vi "FPGAmain_5782_IQ_PID.vi"() -> ()   [LabVIEW 2018]
uses:
  FPGA/DataMode.ctl
  FPGA/Input_5782/5782_Fast_PID_states.ctl
  FPGA/Feed forward/FeedForwardState.ctl
  FPGA/Feed forward/FeedForwardProcessingState.ctl
  <vilib>/Platform/TimedLoop/XDataNode/timing_clust.ctl
  <vilib>/Platform/TimedLoop/XDataNode/nitl_modes.ctl
  <vilib>/Platform/TimedLoop/XDataNode/wakeup.ctl
  <vilib>/rvi/Emulation/niFpgaSctlEmulationGetInTimedLoop.vi
  <vilib>/rvi/Emulation/niFpgaEmulationReportErrorSimple.vi
  <vilib>/rvi/Emulation/niFpgaGetClockAttributes.vi
  <vilib>/rvi/Emulation/niFpgaCriticalErrorInLSC.vi
  <vilib>/rvi/Emulation/niFpgaProcessEmulError.vi
  <vilib>/rvi/Emulation/niFpgaEmulationIsFPGAContextNoSignature.vi
  <vilib>/rvi/errors/niFpgaSetErrorForExecOnDevCompSimple.vi
  <vilib>/rvi/eio/common/nirviEmuReportErrorAndStop.vi
  <vilib>/rvi/DataTransferAndStorage/Container/Common/niFpgaContainerGetUniqueNameForEmu.vi
  <vilib>/rvi/FIFO/Fifo_Resource/nirvififoEmulationSetSize.vi
  <vilib>/rvi/FIFO/Fifo_Resource/nirviFifoEmulationQueueMgr.vi
  <instcachedir>/0/nirviFifoEmulationQueueMgr_E5CAEC123FF24DC58D834DCA3CDAA9B5.lvgen/nirviFifoEmulationQueueMgr_E5CAEC123FF24DC58D834DCA3CDAA9B5_015.vi
  <vilib>/rvi/FIFO/Fifo_Resource/nirvififoEmulationDetermineInputValidOut.vi
  <vilib>/rvi/FIFO/Fifo_Resource/nirvififoEmulationCreateLock.vi
  <vilib>/rvi/FIFO/Fifo_Resource/nirvififoEmulationObtainLock.vi
  <vilib>/rvi/FIFO/Fifo_Resource/nirvififoEmulationReleaseLock.vi
  <vilib>/rvi/occurrence/nirviWaitOnOccurrenceBase.vi
  <vilib>/rvi/errors/nirviReportUnexpectedCaseInternalError.vi
  <vilib>/rvi/errors/nirviReportUnexpectedCaseInternalError (U32).vi
  <vilib>/rvi/Memory/Memory_Emulation/niFpgaMemoryEmulationCacheClearOnFirstRun.vi
  <vilib>/rvi/Memory/Memory_Emulation/nirvimemoryEmulationManagerCache_MakeExclusive.vi
  <vilib>/rvi/Memory/Memory_Emulation/niFpgaMemoryEmulationValidateCache.vi
  <vilib>/rvi/Memory/Memory_Emulation/nirvimemoryEmulationManagerCache_InsertValue.vi
  <vilib>/Utility/error.llb/Clear Errors.vi
  <vilib>/rvi/Memory/Memory_Emulation/nirvimemoryEmulationManagerCache_ReleaseExclusive.vi
  <vilib>/rvi/Memory/Memory_Emulation/nirvimemoryEmulationManagerCache_GetValue.vi
  <vilib>/rvi/Memory/Memory_Emulation/nirvimemoryEmulationManagerCache_SetValue.vi
  <vilib>/rvi/eio/common/nirviEmuTemplateMethod_errors.vi
  <instcachedir>/0/nirviFifoEmulationQueueMgr_E5CAEC123FF24DC58D834DCA3CDAA9B5.lvgen/nirviFifoEmulationQueueMgr_E5CAEC123FF24DC58D834DCA3CDAA9B5_018.vi
  <vilib>/rvi/interface/RandomDataEmulation/niFpgaRandomDataHandleErrors.vi
  <instcachedir>/0/nirviFifoEmulationQueueMgr_E5CAEC123FF24DC58D834DCA3CDAA9B5.lvgen/nirviFifoEmulationQueueMgr_E5CAEC123FF24DC58D834DCA3CDAA9B5_003.vi
  <instcachedir>/0/nirviFifoEmulationQueueMgr_E5CAEC123FF24DC58D834DCA3CDAA9B5.lvgen/nirviFifoEmulationQueueMgr_E5CAEC123FF24DC58D834DCA3CDAA9B5_017.vi
  <vilib>/rvi/interface/RandomDataEmulation/nirviRandomDataMultiElementFPGAFIFO.vi
  <instcachedir>/0/nirviRandomDataMultiElementFPGAFIFO_6740B454F3C245F78F76ED91F73FD8DB.lvgen/nirviRandomDataMultiElementFPGAFIFO_6740B454F3C245F78F76ED91F73FD8DB_000.vi
  <instrlib>/_niInstr/Basic Elements/v1/FPGA/Private/Count Down U8.vi
  <vilib>/rvi/Memory/Memory_Emulation/nirvimemoryFastEmulation.vi
  <vilib>/rvi/Memory/Memory_Emulation/nirvimemoryEmulation.vi
  <vilib>/Platform/TimedLoop/XDataNode/XDataNode.xnode
  <vilib>/rvi/FXPMathLib/FxpInterpret/XNode/nifxpmath_Interpret.xnode
  <vilib>/rvi/DataTransferAndStorage/Container/XNode/niFpgaContainer.xnode
  <vilib>/rvi/FIFO/Fifo_Resource/nirvififoEmulationWrite.vi
  <vilib>/rvi/DataTransferAndStorage/Register/Emulation/niFpgaRegisterEmulation.vi
  <vilib>/eio/EIONode/EIONode.xnode
  <vilib>/rvi/FIFO/Fifo_Resource/nirvififoEmulationRead.vi
  <vilib>/rvi/interface/RandomDataEmulation/nirviRandomDataFpgaReadWriteTemplate.vi
  <vilib>/rvi/interface/RandomDataEmulation/nirviRandomDataFpgaMultiElementTemplate.vi
  <vilib>/Platform/TimedLoop/XDataNode/XDNodeRunTimeDep.lvlib
  <instrlib>/_niInstr/Basic Elements/v1/FPGA/niInstr Basic Elements v1 FPGA.lvlib
panel:
  in  "Ultra low speed transfer":bool
  out "5782 states":T1
  out "Read FF address":u32
  in  "Load FF":bool
  in  "Clear feedback buffers":bool
  in  "FF buffers manual":bool
  in  "Full speed transfer":bool
  in  "IO Module\\AO Data Sync":bool=TRUE
  in  "IO Module\\SPI Write Data":u16
  out "IO Module\\SPI Read Data":u8
  in  "IO Module\\SPI Read":bool
  in  "IO Module\\SPI Write":bool
  in  "IO Module\\SPI Address":u16
  in  "IO Module\\SPI Device":u8
  out "IO Module\\SPI Idle":bool
  in  "AM phase":fxp<+,64,64>
  in  "User Command Commit":bool
  in  "User Command":u8
  out "User Command Idle":bool
  out "User Command Status":u8
  in  "User Data 0":u8
  in  "User Data 1":u8
  out "PLL Locked":bool
  out "User Error":bool
  out "Configured?":bool
  in  "Continuous":bool
  in  "Record length":u16=4000 caption="Samples Per Trigger" min=1 step=1
  in  "Trigger Acquisition":bool
  out "IO Module\\Trigger Input":bool
  in  "Acquisition running":bool
  in  "Phase output":fxp<+,64,64>[](array[numeric])=[0.0, 0.0, 0.0, 0.0]
  in  "Simulated phase":fxp<+,64,64>[](array[numeric])=[0.0, 0.0]
  in  "Mode":T2
  in  "Phase input":fxp<+,64,64>[](array[numeric])=[0.0, 0.0, 0.0, 0.0, 0.0, 0.0, 0.0, 0.0, 0.0, 0.0, 0.0, 0.0, 0.0, 0.0, 0.0, 0.0]
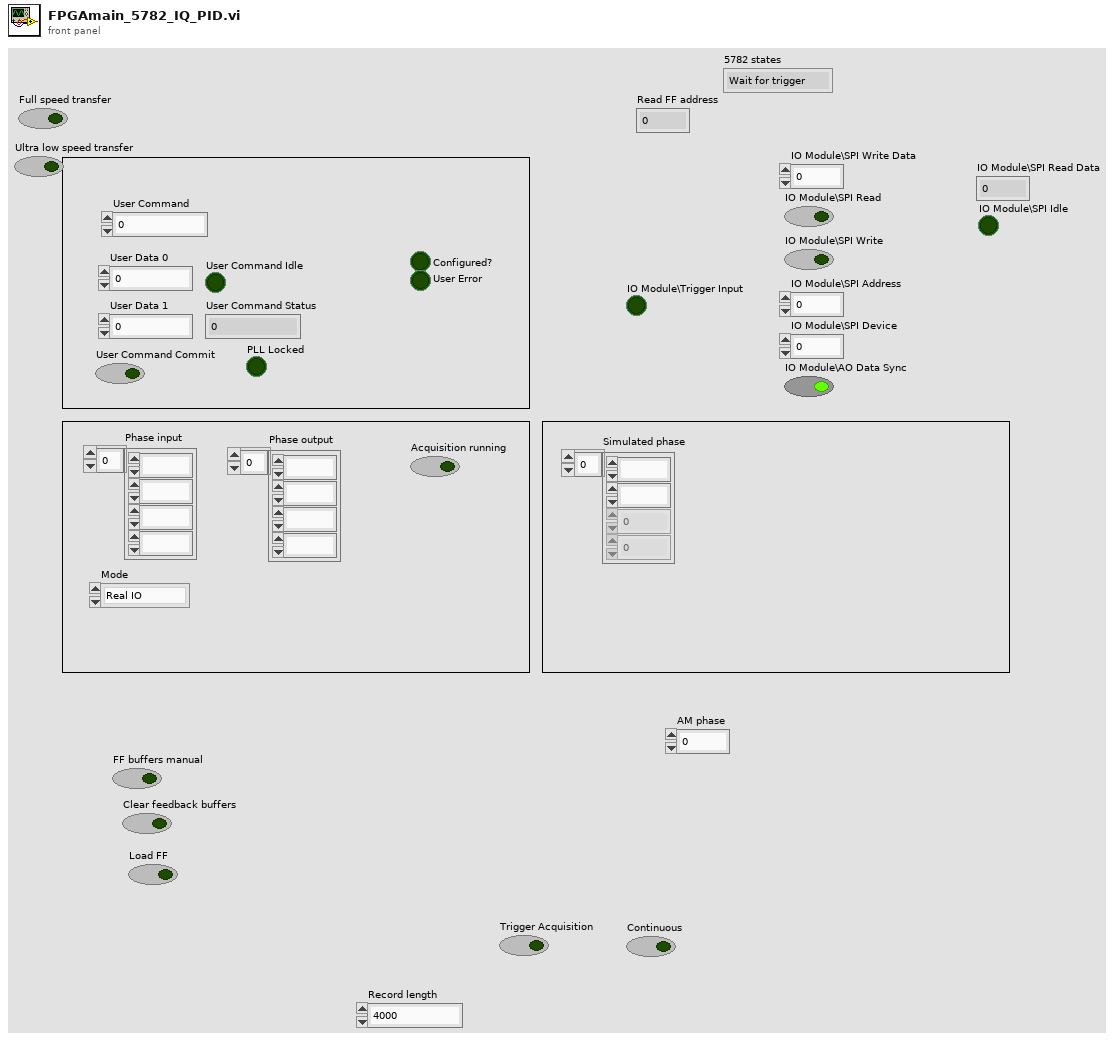
[diagram p1: front panel]
types:
  T1 = typedef "5782_Fast_PID_states.ctl" = enum8{"Wait for trigger", "Acquisition", "Send record length", "Wait for output", "Quiet period"}
  T2 = typedef "DataMode.ctl" = enum16{"Real IO", "Simulated"}
  T3 = typedef "FeedForwardProcessingState.ctl" = enum16{"Wait for trigger", "Processing", "Filtering", "Wait for reset"}
  T4 = typedef "FeedForwardState.ctl" = enum16{"Idle", "Wait for trigger", "Read FF", "Clear FF", "Wait for reset"}
  T5 = typedef "XDNodeRunTimeDep.lvlib/timing_clust.ctl" = cluster{"Expected End [f-1]":u64, "Actual End [f-1]":u64, "Finished Late? [f-1]":bool, "Expected End [i-1]":u64, "Actual End [i-1]":u64, "Finished Late? [i-1]":bool, "Expected Start [i]":u64, "Actual Start [i]":u64, "Expected Start [f]":u64, "Actual Start [f]":u64, "Source Name":string, "Structure Name":string, "Period":i64, "Deadline":i64, "Offset":i64, "Start":i64, "Priority":i32, "Timeout":i32, "Mode":T6, "Wakeup Reason":T7, "Error":errorcluster, "Source Type":string, "Secondary Source Type":string, "Global End Time":u64, "Global Start Time":u64, "Frame Duration":u64, "Iteration Duration":u64, "Assigned CPU":i32, "I/O Scan Engine Mode":u32}
  T6 = typedef "XDNodeRunTimeDep.lvlib/nitl_modes.ctl" = enum32{"No Change", "Process missed periods, maintain original phase", "Discard missed periods, maintain original phase", "Process missed periods, ignore original phase", "Discard missed periods, ignore original phase"}
  T7 = typedef "XDNodeRunTimeDep.lvlib/wakeup.ctl" = enum32{"Normal", "Aborted", "Asynchronous wakeup", "Timing source error", "Timed loop error", "Timeout"}
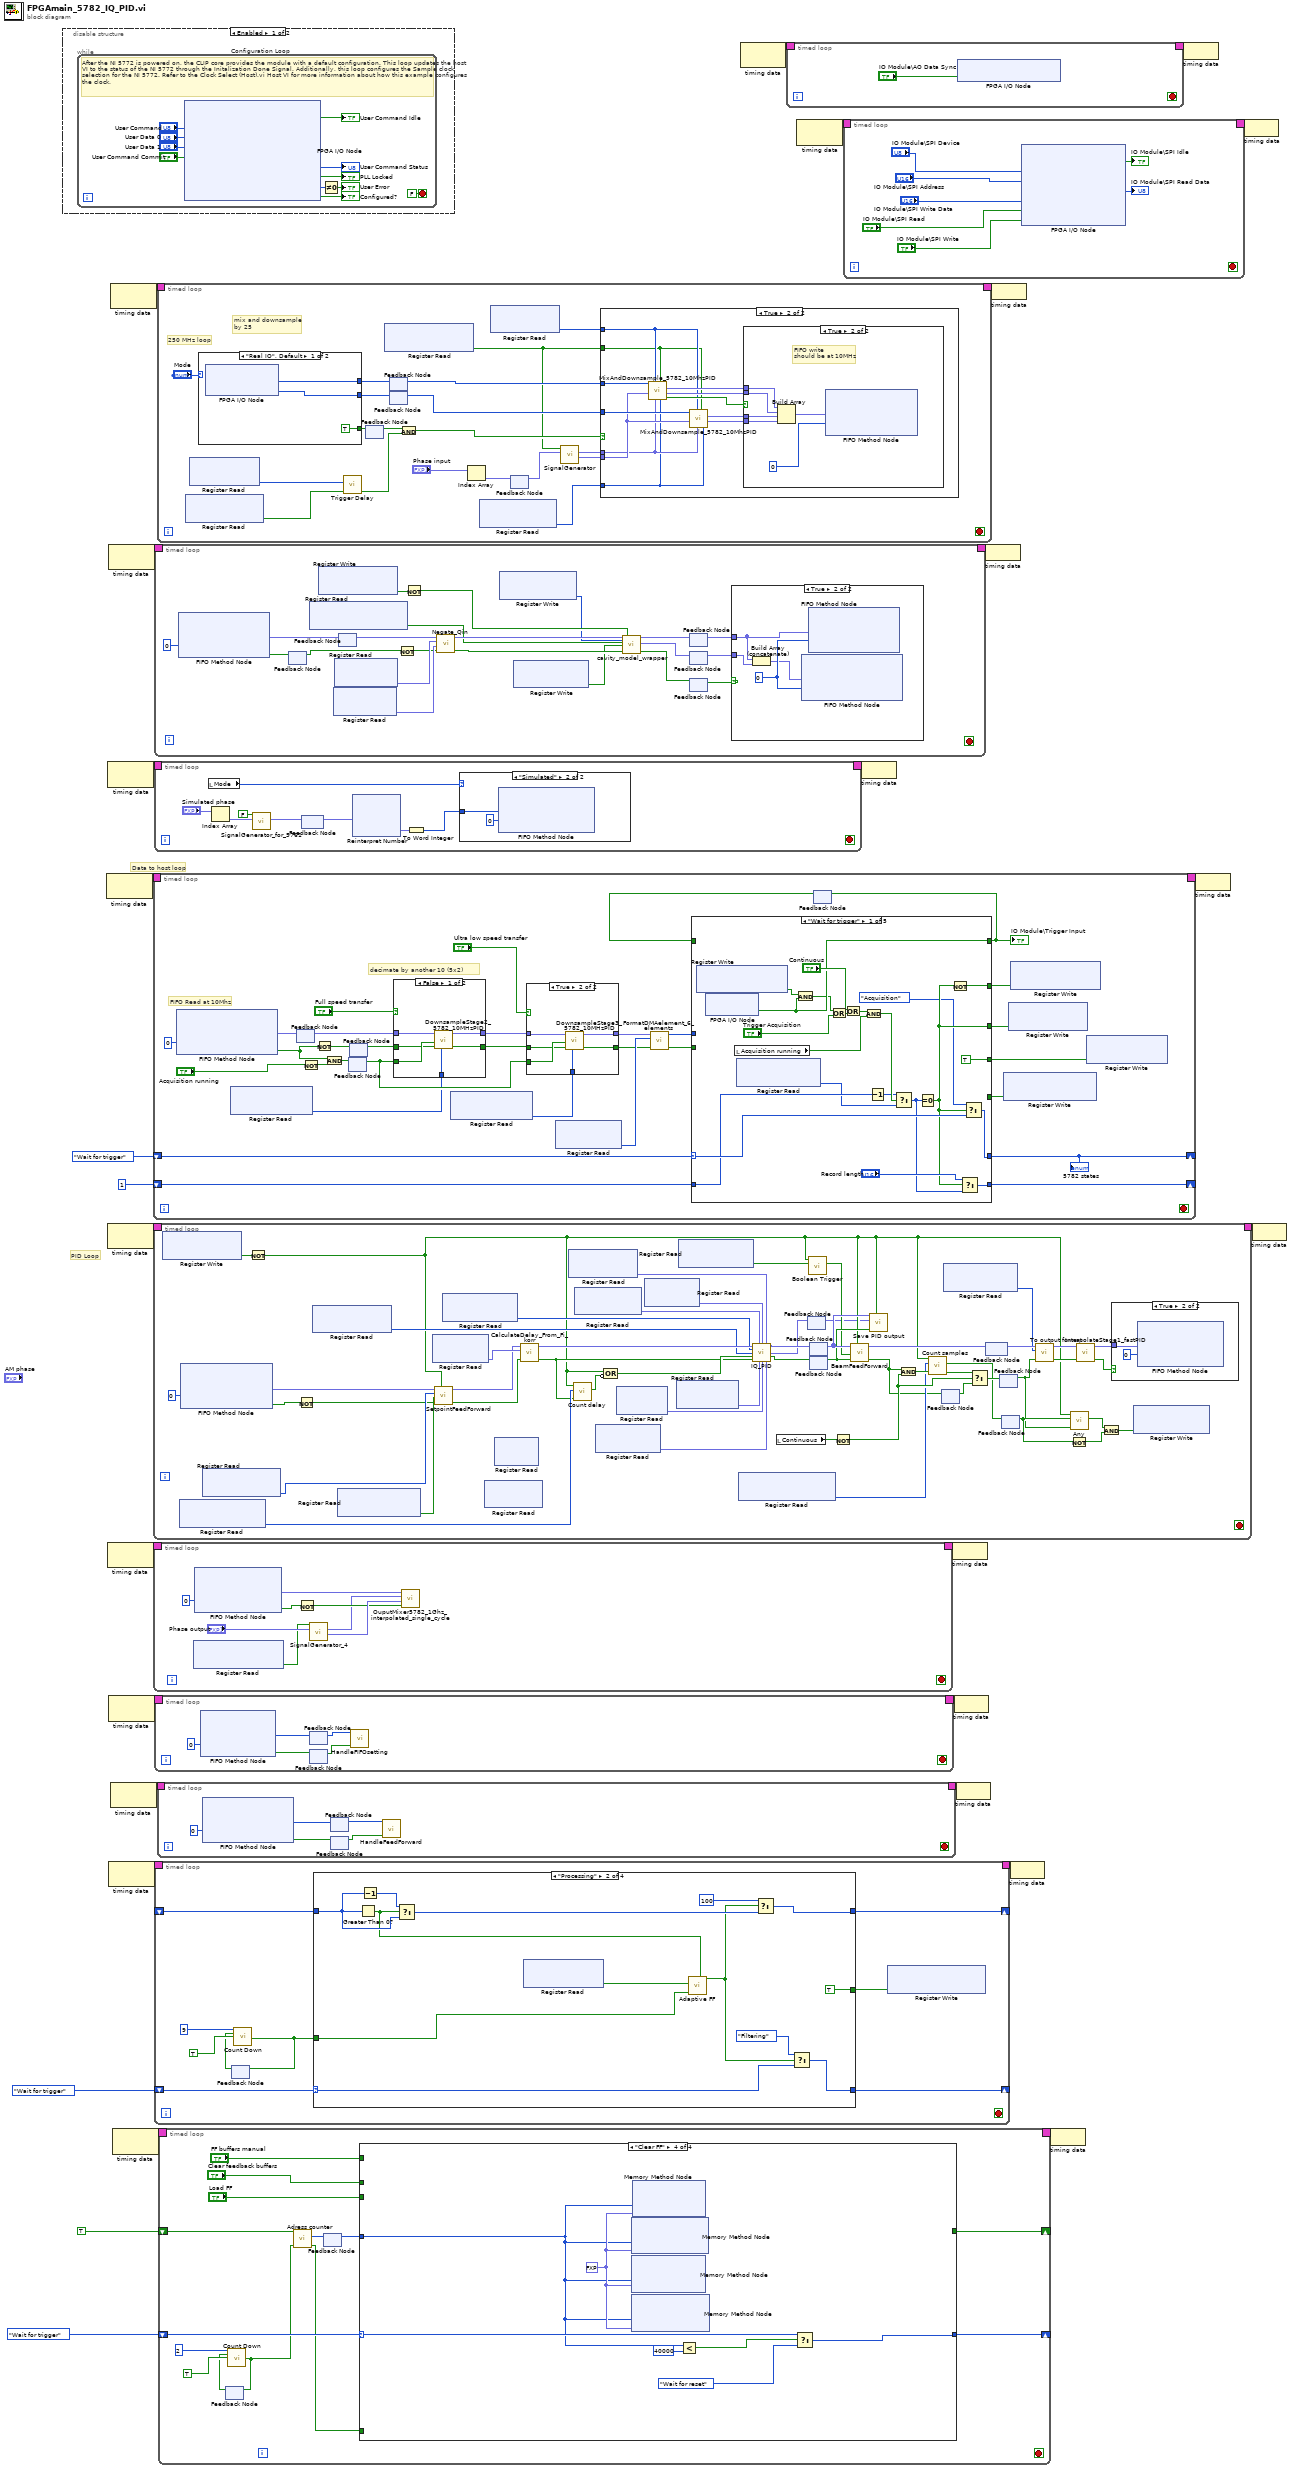
[diagram p0: block diagram]
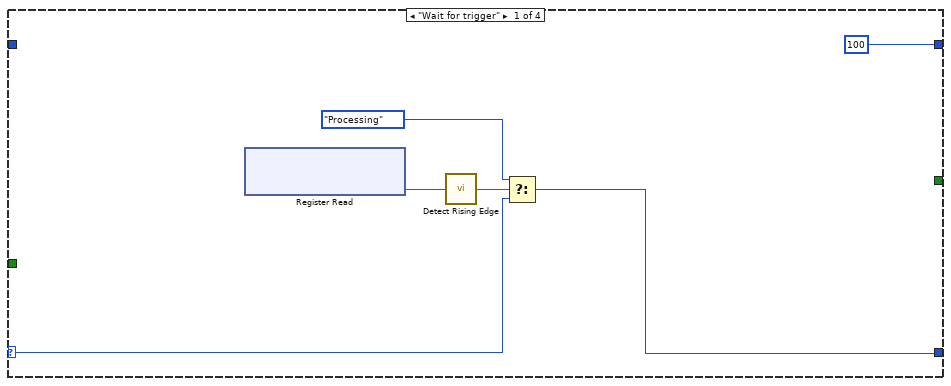
[diagram p2: hidden frame]
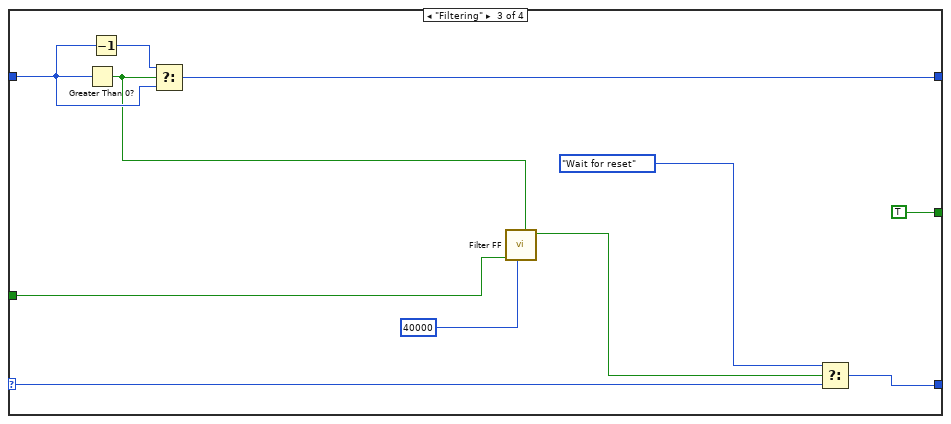
[diagram p3: hidden frame]
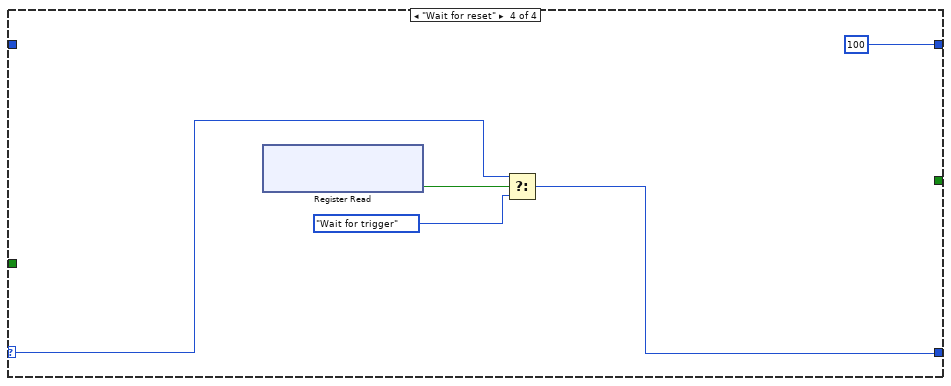
[diagram p4: hidden frame]
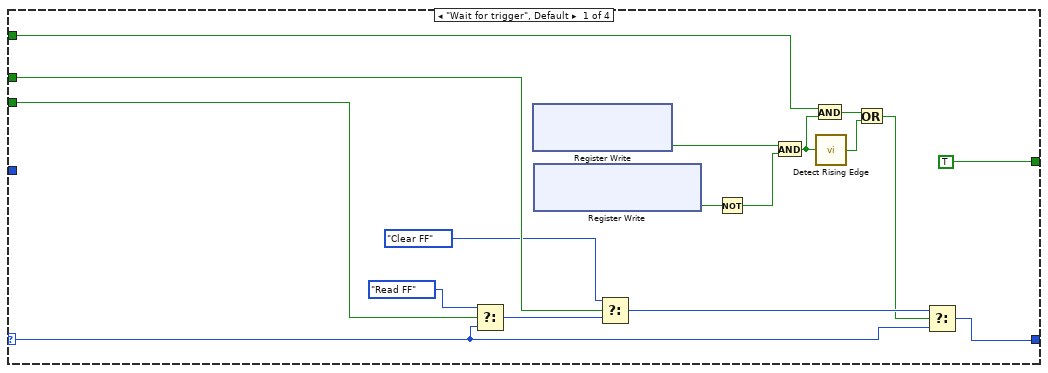
[diagram p5: hidden frame]
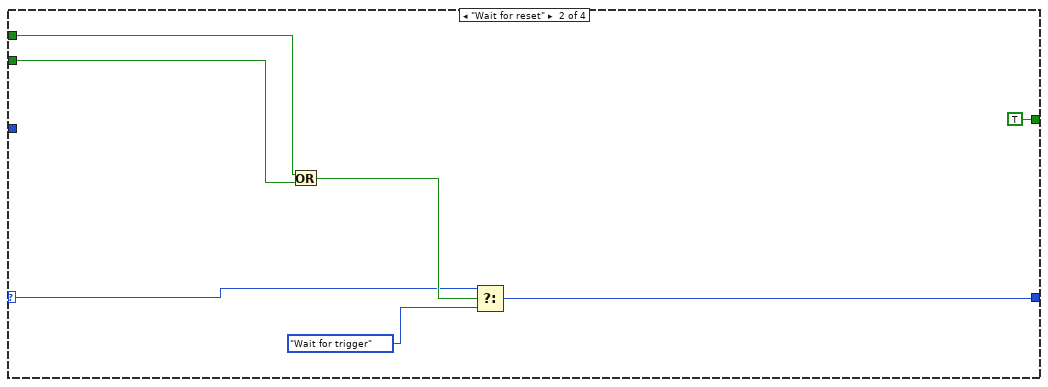
[diagram p6: hidden frame]
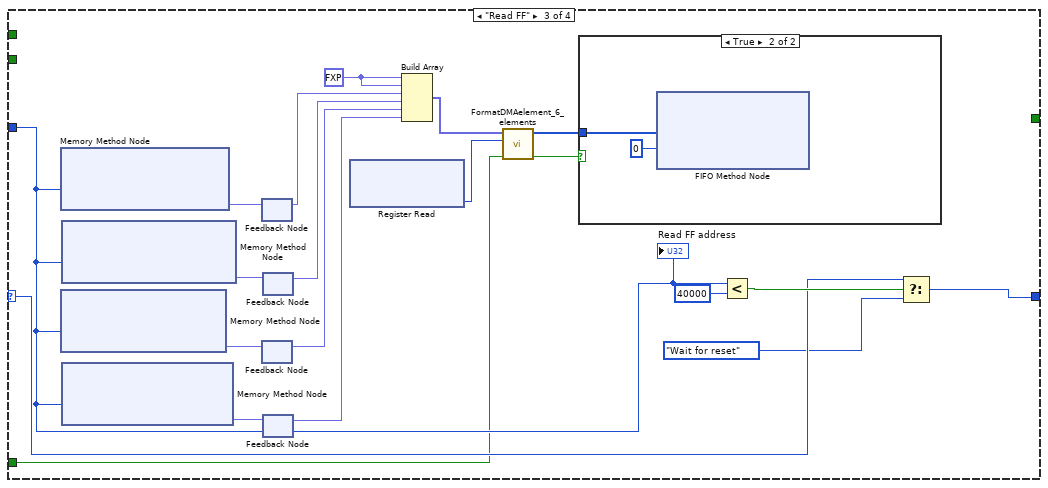
[diagram p7: hidden frame]
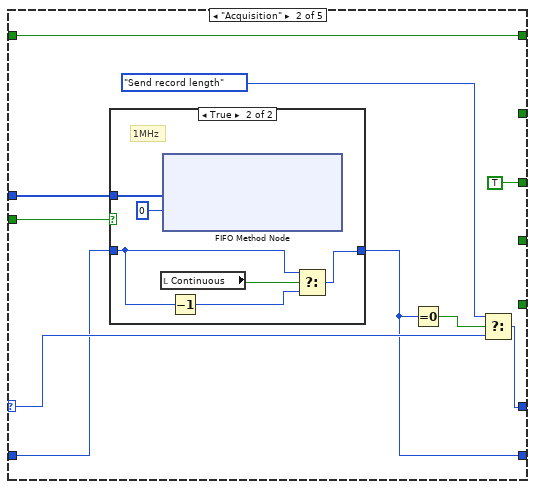
[diagram p12: hidden frame]
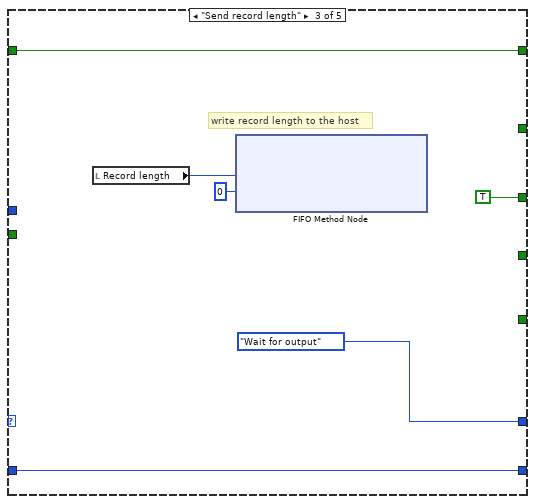
[diagram p14: hidden frame]
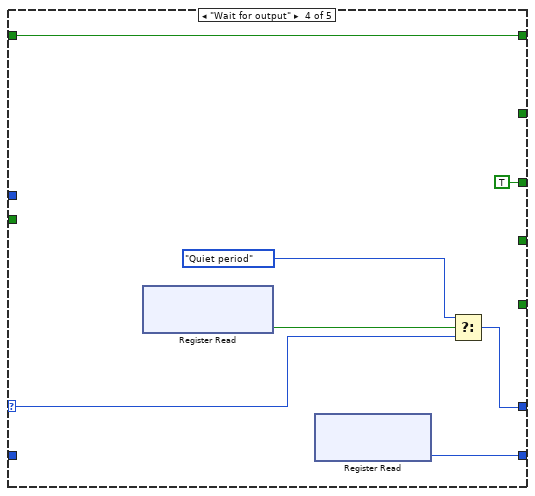
[diagram p15: hidden frame]
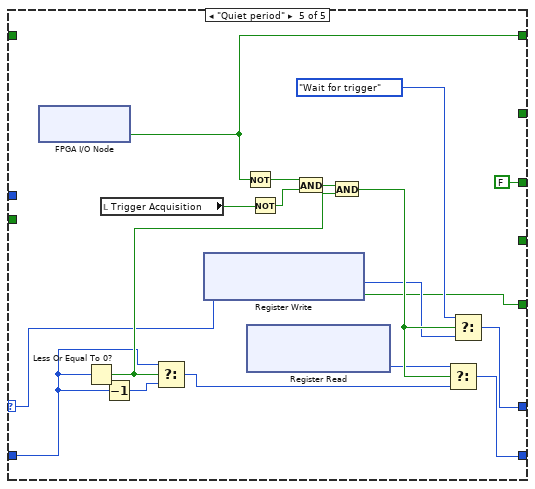
[diagram p16: hidden frame]
diagram:
  # "PID Loop"
  # "Data to host loop"
  n1 = disable-structure shown="Enabled" {
    frame Enabled {
      n2 = while "Configuration Loop" {
        stop <- FALSE stop-if-true
        # "After the NI 5772 is powered on, the CLIP core provides the module with a default configuration. This loop updates the host VI to the status of the NI 5772 through the Initalization Done Signal. Additionally, this loop configures the Sample clock selection for the NI 5772. Refer to the Clock Select (Host).vi Host VI for more information about how this example configures the clock."
        n3 = xnode "FPGA I/O Node"("IO Module\\User Command"="User Command", "IO Module\\User Data 0"="User Data 0", "IO Module\\User Data 1"="User Data 1", "IO Module\\User Command Commit"="User Command Commit") -> ("IO Module\\User Command Idle"=→"User Command Idle":bool, "IO Module\\User Command Status"=→"User Command Status":u8, "IO Module\\PLL Locked"=→"PLL Locked":bool, "IO Module\\User Error"=w35:u8, "IO Module\\Initialization Done"=→"Configured?":bool)  [unwired: 9 in, 9 out]
        n4 = Not Equal To 0?(x=w35) -> (x != 0?=→"User Error":bool)
      }
    }
    frame Disabled {
    }
  }
  n5 = node-c288() -> (w14:T5)  [unwired: 1 in]
  n6 = node-c288() -> (w16:T5)  [unwired: 1 in]
  n7 = node-c288() -> (w22:T5)  [unwired: 1 in]
  n8 = node-c288() -> (w29:T5)  [unwired: 1 in]
  n9 = node-c288() -> (w9:T5)  [unwired: 1 in]
  n10 = node-c288() -> (w24:T5)  [unwired: 1 in]
  n11 = node-c288() -> (w3:T5)  [unwired: 1 in]
  n12 = node-c288() -> (w27:T5)  [unwired: 1 in]
  n13 = node-c288() -> (w11:T5)  [unwired: 1 in]
  n14 = node-c288() -> (w7:T5)  [unwired: 1 in]
  n15 = timed-loop {
    timing: w14 -> [_]
    timing-out: [_] -> w13
    shift-right: [w69] -> _
    shift-left: 5782_Fast_PID_states."Wait for trigger" ("5782 states") -> [w71]
    shift-right: [w68] -> _
    shift-left: u16 1 ("trigger samples") -> [w70]
    stop <- _ stop-if-true
    # "FIFO Read at 10Mhz"
    # "decimate by another 10 (5x2)"
    n16 = xnode ("FIFO Method Node")("Timeout"=0) -> ("Element"=w51:fxp<+/-,32,14>[], "Timed Out?"=w50:bool)  [unwired: 1 in, 1 out]
    n17 = xnode ("Register Read")() -> ("Data"=w42:u32)  [unwired: 1 in, 1 out]
    n18 = feedback #1() -> (w52:fxp<+/-,32,14>[])  [unwired: 1 in]
    n19 = feedback-in #1(w51) -> ()
    n20 = Not(x="Acquisition running") -> (.not. x?=w57:bool)
    n21 = Not(x=w50) -> (.not. x?=w55:bool)
    n22 = And(x=w50, y=w57) -> (x .and. y?=w54:bool)
    n23 = feedback #2() -> (w47:bool)  [unwired: 1 in]
    n24 = feedback-in #2(w54) -> ()
    n25 = feedback #3() -> (w56:bool)  [unwired: 1 in]
    n26 = feedback-in #3(w55) -> ()
    n27 = case shown="False" "Full speed transfer" {
      tunnel: [w85 w87] -> w45
      tunnel: [w84 w86] -> w46
      tunnel: w52 -> [w83 w87]
      tunnel: w47 -> [w82 _]
      tunnel: w56 -> [w81 w86]
      tunnel: w42 -> [w80 _]
      frame False {
        n28 = call "DownsampleStage2_5782_10MHzPID.vi"("Count to skip"=w80, "valid in"=w81, "reset"=w82, "Data in"=w83) -> ("valid out"=w84:bool, "data out"=w85:fxp<+/-,32,14>[])  [unwired: 6 in]
      }
      frame True {
      }
    }
    n29 = xnode ("Register Read")() -> ("Data"=w41:u32)  [unwired: 1 in, 1 out]
    n30 = case shown="True" "Ultra low speed transfer" {
      tunnel: [w73 w78] -> w43
      tunnel: [w72 w77] -> w44
      tunnel: w45 -> [w73 w79]
      tunnel: w47 -> [_ w76]
      tunnel: w46 -> [w72 w75]
      tunnel: w41 -> [_ w74]
      frame False {
      }
      frame True {
        n31 = call "DownsampleStage3_5782_10MHzPID.vi"("Count to skip"=w74, "valid in"=w75, "reset"=w76, "Data in"=w79) -> ("valid out"=w77:bool, "data out"=w78:fxp<+/-,32,14>[])  [unwired: 6 in]
      }
    }
    n32 = xnode ("Register Read")() -> ("Data"=w61:u16)  [unwired: 1 in, 1 out]
    n33 = call "FormatDMAelement_6_elements.vi"("valid in"=w44, "factor"=w61, "Data in"=w43) -> ("valid out"=w64:bool, "Values"=w63:u64[])  [unwired: 7 in]
    n34 = feedback #4() -> (w66:bool)  [unwired: 1 in]
    n35 = case shown="\"Wait for trigger\"" w71 {
      selector: w71 -> [w108 w118 _ w136 w143]
      tunnel: w70 -> [w99 w115 w126 _ w144]
      tunnel: [w107 w117 5782_Fast_PID_states."Wait for output" ("5782 states") w138 w154] -> w69
      tunnel: [w106 w112 w126 w134 w155] -> w68
      tunnel: w63 -> [_ w113 _ _ _]
      tunnel: w64 -> [_ w114 _ _ _]
      tunnel: [w94 TRUE TRUE ("5782 triggered") TRUE ("5782 triggered") FALSE ("5782 triggered")] -> w67
      tunnel: [w89 w111 w128 w133 w139] -> w65
      tunnel: w66 -> [_ w111 w128 w133 _]
      tunnel: [w93 _ _ _ _] -> w62
      tunnel: [TRUE _ _ _ _] -> w60
      tunnel: [_ _ _ _ w141] -> w59
      frame "Wait for trigger" {
        n36 = xnode "Register Write"() -> ("Data"=w90:bool)  [unwired: 1 in, 1 out]
        n37 = xnode "FPGA I/O Node"() -> ("PXI_Trig0"=w89:bool)  [unwired: 1 in, 1 out]
        n38 = local read "Acquisition running"() -> (w102:bool)
        n39 = xnode ("Register Read")() -> ("Data"=w95:u16)  [unwired: 1 in, 1 out]
        n40 = And(x=w90, y=w89) -> (x .and. y?=w88:bool)
        n41 = Or(x=w88, y="Trigger Acquisition") -> (x .or. y?=w98:bool)
        n42 = Or(x="Continuous", y=w98) -> (x .or. y?=w96:bool)
        n43 = And(x=w96, y=w102) -> (x .and. y?=w103:bool)
        n44 = Decrement(x=w99) -> (x-1=w100:u16)
        n45 = Select(t=w100, s=w103, f=w95) -> (s? t:f=w101:u16)
        n46 = Equal To 0?(x=w101) -> (x = 0?=w94:bool)
        n47 = Not(x=w94) -> (.not. x?=w93:bool)
        n48 = Select(t="Record length", s=w94, f=w101) -> (s? t:f=w106:u16)
        n49 = Select(t=5782_Fast_PID_states."Acquisition" ("5782 states"), s=w94, f=w108) -> (s? t:f=w107:T1)
      }
      frame "Acquisition" {
        n50 = case shown="True" w114 {
          tunnel: w113 -> [_ w125]
          tunnel: [w119 w122] -> w112
          tunnel: w115 -> [w119 w120]
          frame False {
          }
          frame True {
            # "1MHz"
            n51 = local read "Continuous"() -> (w123:bool)
            n52 = xnode ("FIFO Method Node")("Element"=w125, "Timeout"=0) -> ()  [unwired: 1 in, 2 out]
            n53 = Decrement(x=w120) -> (x-1=w121:u16)
            n54 = Select(t=w120, s=w123, f=w121) -> (s? t:f=w122:u16)
          }
        }
        n55 = Equal To 0?(x=w112) -> (x = 0?=w116:bool)
        n56 = Select(t=5782_Fast_PID_states."Send record length" ("5782 states"), s=w116, f=w118) -> (s? t:f=w117:T1)
      }
      frame "Send record length" {
        # "write record length to the host"
        n57 = local read "Record length"() -> (w130:u16)
        n58 = xnode ("FIFO Method Node")("Element"=w130, "Timeout"=0) -> ()  [unwired: 1 in, 2 out]
      }
      frame "Wait for output" {
        n59 = xnode ("Register Read")() -> ("Data"=w132:bool)  [unwired: 1 in, 1 out]
        n60 = xnode ("Register Read")() -> ("Data"=w134:u16)  [unwired: 1 in, 1 out]
        n61 = Select(t=5782_Fast_PID_states."Quiet period" ("5782 states"), s=w132, f=w136) -> (s? t:f=w138:T1)
      }
      frame "Quiet period" {
        n62 = xnode "FPGA I/O Node"() -> ("PXI_Trig0"=w139:bool)  [unwired: 1 in, 1 out]
        n63 = Less Or Equal To 0?(x=w144) -> (x <= 0?=w147:bool)
        n64 = local read "Trigger Acquisition"() -> (w152:bool)
        n65 = Decrement(x=w144) -> (x-1=w148:u16)
        n66 = Select(t=w144, s=w147, f=w148) -> (s? t:f=w146:u16)
        n67 = xnode ("Register Write")() -> ("Data"=w141:bool)  [unwired: 1 in, 1 out]
        n68 = Not(x=w139) -> (.not. x?=w140:bool)
        n69 = xnode ("Register Read")() -> ("Data"=w145:u16)  [unwired: 1 in, 1 out]
        n70 = Not(x=w152) -> (.not. x?=w151:bool)
        n71 = And(x=w140, y=w151) -> (x .and. y?=w150:bool)
        n72 = And(x=w150, y=w147) -> (x .and. y?=w153:bool)
        n73 = Select(t=w145, s=w153, f=w146) -> (s? t:f=w155:u16)
        n74 = Select(t=5782_Fast_PID_states."Wait for trigger" ("5782 states"), s=w153, f=w143) -> (s? t:f=w154:T1)
      }
    }
    "IO Module\\Trigger Input" <- w65
    "5782 states" <- w69
    n75 = feedback-in #4(w65) -> ()
    n76 = xnode ("Register Write")("Data"=w59) -> ()  [unwired: 1 in, 1 out]
    n77 = xnode ("Register Write")("Data"=w67) -> ()  [unwired: 1 in, 1 out]
    n78 = xnode ("Register Write")("Data"=w62) -> ()  [unwired: 1 in, 1 out]
    n79 = xnode ("Register Write")("Data"=w60) -> ()  [unwired: 1 in, 1 out]
  }
  n80 = timed-loop {
    timing: w16 -> [_]
    timing-out: [_] -> w15
    stop <- _ stop-if-true
    n81 = xnode ("Register Write")() -> ("Data"=w208:bool)  [unwired: 1 in, 1 out]
    n82 = xnode ("Register Read")() -> ("Data"=w204:u32)  [unwired: 1 in, 1 out]
    n83 = xnode ("FIFO Method Node")("Timeout"=0) -> ("Element"=w202:fxp<+/-,32,14>[], "Timed Out?"=w209:bool)  [unwired: 1 in, 1 out]
    n84 = xnode ("Register Read")() -> ("Data"=w203:u32)  [unwired: 1 in, 1 out]
    n85 = Not(x=w208) -> (.not. x?=w162:bool)
    n86 = Not(x=w209) -> (.not. x?=w201:bool)
    n87 = xnode ("Register Read")() -> ("Data"=w188:enum16{"PID on", "Ref", "Zero"})  [unwired: 1 in, 1 out]
    n88 = xnode ("Register Read")() -> ("Data"=w207:bool)  [unwired: 1 in, 1 out]
    n89 = xnode ("Register Read")() -> ("Data"=w200:fxp<+/-,32,4>)  [unwired: 1 in, 1 out]
    n90 = call "SetpointFeedForward.vi"("Reset"=w162, "input valid"=w201, "setpoint enabled"=w207, "Samples to skip"=w203, "Data in"=w202) -> ("output valid"=w199:bool, "Data out"=w198:fxp<+/-,32,14>[])  [unwired: 5 in]
    n91 = xnode ("Register Read")() -> ("Data"=w196:enum16{"PID on", "Ref", "Zero"})  [unwired: 1 in, 1 out]
    n92 = xnode ("Register Read")() -> ()  [unwired: 1 in, 2 out]
    n93 = xnode ("Register Read")() -> ()  [unwired: 1 in, 2 out]
    n94 = call "CalculateDelay_From_Fi_korr.vi"("input valid"=w199, "fi_korr"=w200, "Data in"=w198) -> ("output valid"=w189:bool, "Data out"=w197:fxp<+/-,32,14>[])  [unwired: 7 in]
    n95 = xnode ("Register Read")() -> ("Data"=w191:fxp<+/-,32,6>)  [unwired: 1 in, 1 out]
    n96 = call "Count delay.vi"("input valid"=w189, "Count to skip"=w204, "Reset"=w162) -> ("count done?"=w205:bool)  [unwired: 7 in, 1 out]
    n97 = xnode ("Register Read")() -> ("Data"=w195:fxp<+/-,32,6>)  [unwired: 1 in, 1 out]
    n98 = xnode ("Register Read")() -> ("Data"=w185:fxp<+/-,32,6>)  [unwired: 1 in, 1 out]
    n99 = Compound Arithmetic op=OR(w162, invert w205) -> (w190:bool)
    n100 = xnode ("Register Read")() -> ("Data"=w186:fxp<+/-,32,6>)  [unwired: 1 in, 1 out]
    n101 = xnode ("Register Read")() -> ("Data"=w194:fxp<+/-,32,6>)  [unwired: 1 in, 1 out]
    n102 = xnode ("Register Read")() -> ("Data"=w187:fxp<+/-,32,6>)  [unwired: 1 in, 1 out]
    n103 = xnode ("Register Read")() -> ("Data"=w163:bool)  [unwired: 1 in, 1 out]
    n104 = xnode ("Register Read")() -> ("Data"=w175:u32)  [unwired: 1 in, 1 out]
    n105 = call "IQ_PID.vi"("Data in"=w197, "Ki*Tau I"=w195, "Kp I"=w194, "Kd/Tau I"=w191, "Enable I"=w196, "Enable Q"=w188, "Reset"=w190, "input valid"=w189, "Ki*Tau Q"=w187, "Kp Q"=w186, "Kd/Tau Q"=w185) -> ("data out"=w193:fxp<+/-,32,14>[], "e(n) out"=w159:fxp<+/-,32,14>[], "output valid"=w192:bool)  [unwired: 2 in]
    n106 = local read "Continuous"() -> (w184:bool)
    n107 = feedback #5() -> (w158:fxp<+/-,32,14>[])  [unwired: 1 in]
    n108 = feedback-in #5(w159) -> ()
    n109 = call "Boolean Trigger.vi"("Value"=w163, "Reset"=w162) -> ("Value out"=w161:bool)  [unwired: 9 in]
    n110 = feedback #6() -> (w167:fxp<+/-,32,14>[])  [unwired: 1 in]
    n111 = feedback-in #6(w193) -> ()
    n112 = feedback #7() -> (w166:bool)  [unwired: 1 in]
    n113 = feedback-in #7(w192) -> ()
    n114 = Not(x=w184) -> (.not. x?=w177:bool)
    n115 = call "BeamFeedForward.vi"("Reset"=w162, "input valid"=w166, "beam enabled"=w161, "Data in"=w167) -> ("output valid"=w164:bool, "Data out"=w165:fxp<+/-,32,14>[])  [unwired: 6 in]
    n116 = call "Save PID output.vi"("Reset"=w162, "input valid"=w166, "e(n) in"=w158, "Data in"=w167) -> ()  [unwired: 8 in]
    n117 = And(x=w164, y=w177) -> (x .and. y?=w179:bool)
    n118 = call "Count samples.vi"("input valid"=w179, "number to count"=w175, "Reset"=w162) -> ("output valid"=w180:bool, "counting"=w176:bool)  [unwired: 7 in]
    n119 = feedback #8() -> (w178:bool)  [unwired: 1 in]
    n120 = feedback-in #8(w164) -> ()
    n121 = xnode ("Register Read")() -> ("Data"=w168:u16)  [unwired: 1 in, 1 out]
    n122 = Select(t=w180, s=w177, f=w178) -> (s? t:f=w181:bool)
    n123 = feedback #9() -> (w172:fxp<+/-,32,14>[])  [unwired: 1 in]
    n124 = feedback-in #9(w165) -> ()
    n125 = feedback-in #10(w181) -> ()
    n126 = feedback #10() -> (w170:bool)  [unwired: 1 in]
    n127 = feedback #11() -> (w183:bool)  [unwired: 1 in]
    n128 = feedback-in #11(w176) -> ()
    n129 = call "To output format.vi"("input valid"=w170, "factor"=w168, "Data in"=w172) -> ("output valid"=w169:bool, "Data out"=w171:fxp<+/-,16,14>[])  [unwired: 7 in]
    n130 = Not(x=w183) -> (.not. x?=w182:bool)
    n131 = call "Any.vi"("input valid"=w170, "Value"=w183, "Reset"=w162) -> ("Any?"=w160:bool)  [unwired: 7 in, 1 out]
    n132 = call "InterpolateStage1_fastPID.vi"("valid in"=w169, "Data in"=w171) -> ("valid out"=w173:bool, "Data out"=w174:fxp<+/-,16,14>[])  [unwired: 8 in]
    n133 = And(x=w160, y=w182) -> (x .and. y?=w206:bool)
    n134 = case shown="True" w173 {
      tunnel: w174 -> [_ w212]
      frame False {
      }
      frame True {
        n135 = xnode ("FIFO Method Node")("Element"=w212, "Timeout"=0) -> ()  [unwired: 1 in, 2 out]
      }
    }
    n136 = xnode ("Register Write")("Data"=w206) -> ()  [unwired: 1 in, 1 out]
  }
  n137 = timed-loop {
    timing: w22 -> [_]
    timing-out: [_] -> w21
    stop <- _ stop-if-true
    n138 = xnode ("Register Read")() -> ("Data"=w215:bool)  [unwired: 1 in, 1 out]
    n139 = xnode ("FIFO Method Node")("Timeout"=0) -> ("Element"=w218:fxp<+/-,16,14>[], "Timed Out?"=w221:bool)  [unwired: 1 in, 1 out]
    n140 = Not(x=w221) -> (.not. x?=w217:bool)
    n141 = call "SignalGenerator_4.vi"("Phase"="Phase output", "reset"=w215) -> ("Sine out"=w219:fxp<+/-,16,0>[], "Cosine out"=w216:fxp<+/-,16,0>[])  [unwired: 8 in]
    n142 = call "OuputMixer5782_1Ghz_interpolated_single_cycle.vi"("input valid"=w217, "Sine in"=w219, "Cosine in"=w216, "Data"=w218) -> ()  [unwired: 7 in, 1 out]
  }
  n143 = timed-loop {
    timing: w29 -> [_]
    timing-out: [_] -> w28
    stop <- _ stop-if-true
    n144 = local read "Mode"() -> (w232:T2)
    n145 = Index Array(array="Simulated phase") -> (element=w231:fxp<+,64,64>)  [unwired: 1 in]
    n146 = call "SignalGenerator_for_5761.vi"("phase"=w231, "Reset"=FALSE) -> ("Sin"=w227:fxp<+/-,16,0>)  [unwired: 7 in, 2 out]
    n147 = feedback #12() -> (w228:fxp<+/-,16,0>)  [unwired: 1 in]
    n148 = feedback-in #12(w227) -> ()
    n149 = xnode "Reinterpret Number"("x"=w228) -> ("y"=w229:fxp<+/-,16,13>)
    n150 = To Word Integer(number=w229) -> (16bit integer=w225:i16)
    n151 = case shown="\"Simulated\"" w232 {
      tunnel: w225 -> [_ w233]
      frame "Real IO", Default {
      }
      frame "Simulated" {
        n152 = xnode ("FIFO Method Node")("Element"=w233, "Timeout"=0) -> ()  [unwired: 1 in, 2 out]
      }
    }
  }
  n153 = timed-loop {
    timing: w9 -> [_]
    timing-out: [_] -> w8
    stop <- _ stop-if-true
    n154 = xnode ("FIFO Method Node")("Timeout"=0) -> ("Element"=w243:fxp<+/-,32,14>[], "Timed Out?"=w242:bool)  [unwired: 1 in, 1 out]
    n155 = feedback #13() -> (w240:bool)  [unwired: 1 in]
    n156 = feedback-in #13(w242) -> ()
    n157 = xnode ("Register Read")() -> ("Data"=w251:bool)  [unwired: 1 in, 1 out]
    n158 = xnode ("Register Write")() -> ("Data"=w250:bool)  [unwired: 1 in, 1 out]
    n159 = xnode ("Register Read")() -> ("Data"=w256:fxp<+/-,32,14>)  [unwired: 1 in, 1 out]
    n160 = xnode ("Register Read")() -> ("Data"=w257:fxp<+/-,32,14>)  [unwired: 1 in, 1 out]
    n161 = feedback #14() -> (w241:fxp<+/-,32,14>[])  [unwired: 1 in]
    n162 = feedback-in #14(w243) -> ()
    n163 = Not(x=w240) -> (.not. x?=w255:bool)
    n164 = Not(x=w250) -> (.not. x?=w252:bool)
    n165 = call "Negate_Qin.vi"("valid in"=w255, "DC offset chan 1"=w256, "DC offset chan 0"=w257, "Data in"=w241) -> ("valid out"=w253:bool, "Data out"=w254:fxp<+/-,32,14>[])  [unwired: 6 in]
    n166 = xnode "Register Write"() -> ("Data"=w237:enum16{"Off", "On - Ch 0", "On - Ch 1"})  [unwired: 1 in, 1 out]
    n167 = xnode "Register Write"() -> ("Data"=w238:bool)  [unwired: 1 in, 1 out]
    n168 = call "cavity_model_wrapper.vi"("Data in"=w254, "Piezo setting"=w237, "enabled"=w251, "virtual cavity"=w238, "input valid"=w253, "reset"=w252) -> ("Data out"=w249:fxp<+/-,32,14>[], "Ai1 out"=w245:fxp<+/-,32,14>[], "output valid"=w247:bool)  [unwired: 11 in]
    n169 = feedback #15() -> (w248:fxp<+/-,32,14>[])  [unwired: 1 in]
    n170 = feedback-in #15(w249) -> ()
    n171 = feedback #16() -> (w244:fxp<+/-,32,14>[])  [unwired: 1 in]
    n172 = feedback-in #16(w245) -> ()
    n173 = feedback #17() -> (w246:bool)  [unwired: 1 in]
    n174 = feedback-in #17(w247) -> ()
    n175 = case shown="True" w246 {
      tunnel: w248 -> [_ w260]
      tunnel: w244 -> [_ w259]
      frame False {
      }
      frame True {
        w261 = 0 ("Timeout")
        n176 = Build Array (concatenate)(w260, w259) -> (w258:fxp<+/-,32,14>[])
        n177 = xnode ("FIFO Method Node")("Element"=w258, "Timeout"=w261) -> ()  [unwired: 1 in, 2 out]
        n178 = xnode ("FIFO Method Node")("Element"=w260, "Timeout"=w261) -> ()  [unwired: 1 in, 2 out]
      }
    }
  }
  n179 = timed-loop {
    timing: w24 -> [_]
    timing-out: [_] -> w23
    stop <- _ stop-if-true
    n180 = xnode ("FIFO Method Node")("Timeout"=0) -> ("Element"=w267:u64, "Timed Out?"=w266:bool)  [unwired: 1 in, 1 out]
    n181 = feedback #18() -> (w265:u64)  [unwired: 1 in]
    n182 = feedback-in #18(w267) -> ()
    n183 = feedback #19() -> (w264:bool)  [unwired: 1 in]
    n184 = feedback-in #19(w266) -> ()
    n185 = call "HandleFIFOsetting.vi"("timed out"=w264, "Value"=w265) -> ()  [unwired: 10 in]
  }
  n186 = timed-loop {
    timing: w3 -> [_]
    timing-out: [_] -> w2
    shift-right: [w274] -> _
    shift-left: FeedForwardProcessingState."Wait for trigger" ("Processing state") -> [w275]
    shift-right: [w272] -> _
    shift-left: _ -> [w273]
    stop <- _ stop-if-true
    n187 = feedback #20() -> (w277:bool)  [unwired: 1 in]
    n188 = call-poly <instrlib>:"Count Down.vi"("count in"=u8 9, "load"=w277, "decrement"=TRUE) -> ("terminal count"=w276:bool)  [unwired: 11 in, 1 out]
    n189 = feedback-in #20(w276) -> ()
    n190 = case shown="\"Processing\"" w275 {
      selector: w275 -> [w284 w291 w305 w313]
      tunnel: w276 -> [_ w287 w301 _]
      tunnel: [w283 w289 w303 w312] -> w274
      tunnel: w273 -> [_ w297 w308 _]
      tunnel: [u8 100 ("unsigned 8bit integer") w293 w299 u8 100 ("unsigned 8bit integer")] -> w272
      tunnel: [_ TRUE ("Data") TRUE ("Data") _] -> w271
      frame "Wait for trigger" {
        n191 = xnode ("Register Read")() -> ("Data"=w281:bool)  [unwired: 1 in, 1 out]
        n192 = call <instrlib>:"Detect Rising Edge.vi"("signal"=w281) -> ("edge detected"=w280:bool)  [unwired: 14 in]
        n193 = Select(t=FeedForwardProcessingState."Processing" ("Processing state"), s=w280, f=w284) -> (s? t:f=w283:T3)
      }
      frame "Processing" {
        n194 = Greater Than 0?(x=w297) -> (x > 0?=w296:bool)
        n195 = Decrement(x=w297) -> (x-1=w298:u8)
        n196 = Select(t=w298, s=w296, f=w297) -> (s? t:f=w294:u8)
        n197 = xnode "Register Read"() -> ("Data"=w286:bool)  [unwired: 1 in, 1 out]
        n198 = call "Adaptive FF.vi"("Reset"=w296, "input valid"=w287, "Disable e(n)"=w286) -> ("done"=w292:bool)  [unwired: 7 in, 1 out]
        n199 = Select(t=u8 100 ("s? t:f"), s=w292, f=w294) -> (s? t:f=w293:u8)
        n200 = Select(t=FeedForwardProcessingState."Filtering", s=w292, f=w291) -> (s? t:f=w289:T3)
      }
      frame "Filtering" {
        n201 = Greater Than 0?(x=w308) -> (x > 0?=w307:bool)
        n202 = Decrement(x=w308) -> (x-1=w309:u8)
        n203 = Select(t=w309, s=w307, f=w308) -> (s? t:f=w299:u8)
        n204 = call "Filter FF.vi"("Reset"=w307, "Elements in buffer"=u32 40000, "input valid"=w301) -> ("done"=w306:bool)  [unwired: 7 in, 1 out]
        n205 = Select(t=FeedForwardProcessingState."Wait for reset", s=w306, f=w305) -> (s? t:f=w303:T3)
      }
      frame "Wait for reset" {
        n206 = xnode ("Register Read")() -> ("Data"=w310:bool)  [unwired: 1 in, 1 out]
        n207 = Select(t=w313, s=w310, f=FeedForwardProcessingState."Wait for trigger" ("Processing state")) -> (s? t:f=w312:T3)
      }
    }
    n208 = xnode ("Register Write")("Data"=w271) -> ()  [unwired: 1 in, 1 out]
  }
  n209 = timed-loop {
    timing: w27 -> [_]
    timing-out: [_] -> w26
    stop <- _ stop-if-true
    # "mix and downsample\nby 25"
    # "250 MHz loop"
    n210 = xnode ("Register Read")() -> ("Data"=w322:bool)  [unwired: 1 in, 1 out]
    n211 = xnode ("Register Read")() -> ("Data"=w320:u32)  [unwired: 1 in, 1 out]
    n212 = case shown="\"Real IO\", Default" "Mode" {
      tunnel: [w356 w357] -> w334
      tunnel: [w355 w357] -> w332
      tunnel: [TRUE w358] -> w330
      frame "Real IO", Default {
        n213 = xnode "FPGA I/O Node"() -> ("IO Module\\AI 0"=w356:i16, "IO Module\\AI 1"=w355:i16)  [unwired: 2 in, 2 out]
      }
      frame "Simulated" {
        n214 = xnode ("FIFO Method Node")("Timeout"=0) -> ("Element"=w357:i16, "Timed Out?"=w359:bool)  [unwired: 1 in, 1 out]
        n215 = Not(x=w359) -> (.not. x?=w358:bool)
      }
    }
    n216 = call "Trigger Delay.vi"("input valid"=w322, "Count to skip"=w320) -> ("output valid"=w321:bool)  [unwired: 9 in]
    n217 = feedback #21() -> (w329:bool)  [unwired: 1 in]
    n218 = feedback-in #21(w330) -> ()
    n219 = xnode ("Register Read")() -> ("Data"=w318:bool)  [unwired: 1 in, 1 out]
    n220 = feedback #22() -> (w333:i16)  [unwired: 1 in]
    n221 = feedback-in #22(w334) -> ()
    n222 = feedback #23() -> (w331:i16)  [unwired: 1 in]
    n223 = feedback-in #23(w332) -> ()
    n224 = And(x=w329, y=w321) -> (x .and. y?=w326:bool)
    n225 = Index Array(array="Phase input") -> (element=w324:fxp<+,64,64>)  [unwired: 1 in]
    n226 = xnode ("Register Read")() -> ("Data"=w317:u32)  [unwired: 1 in, 1 out]
    n227 = xnode ("Register Read")() -> ("Data"=w319:u16)  [unwired: 1 in, 1 out]
    n228 = feedback #24() -> (w323:fxp<+,64,64>)  [unwired: 1 in]
    n229 = feedback-in #24(w324) -> ()
    n230 = call "SignalGenerator.vi"("phase"=w323, "Reset"=w318) -> ("Cos"=w328:fxp<+/-,16,0>, "Sin"=w327:fxp<+/-,16,0>)  [unwired: 7 in, 1 out]
    n231 = case shown="True" w326 {
      tunnel: w333 -> [_ w347]
      tunnel: w331 -> [_ w346]
      tunnel: w328 -> [_ w340]
      tunnel: w327 -> [_ w339]
      tunnel: w319 -> [_ w338]
      tunnel: w318 -> [_ w337]
      tunnel: w317 -> [_ w336]
      frame False {
      }
      frame True {
        n232 = call "MixAndDownsample_5782_10MhzPID.vi"("Count to skip"=w336, "reset"=w337, "sin0"=w339, "factor"=w338, "cos0"=w340, "signal 0"=w347) -> ("data valid"=w343:bool, "Q out"=w344:fxp<+/-,32,14>, "I out"=w345:fxp<+/-,32,14>)  [unwired: 3 in]
        n233 = call "MixAndDownsample_5782_10MhzPID.vi"("Count to skip"=w336, "reset"=w337, "sin0"=w339, "factor"=w338, "cos0"=w340, "signal 0"=w346) -> ("Q out"=w341:fxp<+/-,32,14>, "I out"=w342:fxp<+/-,32,14>)  [unwired: 3 in, 1 out]
        n234 = case shown="True" w343 {
          tunnel: w344 -> [_ w353]
          tunnel: w345 -> [_ w352]
          tunnel: w342 -> [_ w351]
          tunnel: w341 -> [_ w350]
          frame False {
          }
          frame True {
            # "FIFO write\nshould be at 10MHz"
            n235 = Build Array(w352, w353, w351, w350) -> (w349:fxp<+/-,32,14>[])
            n236 = xnode ("FIFO Method Node")("Element"=w349, "Timeout"=0) -> ()  [unwired: 1 in, 2 out]
          }
        }
      }
    }
  }
  n237 = timed-loop {
    timing: w11 -> [_]
    timing-out: [_] -> w10
    stop <- _ stop-if-true
    n238 = xnode ("FIFO Method Node")("Timeout"=0) -> ("Element"=w366:u64, "Timed Out?"=w364:bool)  [unwired: 1 in, 1 out]
    n239 = feedback #25() -> (w365:u64)  [unwired: 1 in]
    n240 = feedback-in #25(w366) -> ()
    n241 = feedback #26() -> (w363:bool)  [unwired: 1 in]
    n242 = feedback-in #26(w364) -> ()
    n243 = call "HandleFeedForward.vi"("timed out"=w363, "Value"=w365) -> ()  [unwired: 10 in]
  }
  n244 = timed-loop {
    timing: w7 -> [_]
    timing-out: [_] -> w6
    shift-right: [w371] -> _
    shift-left: FeedForwardState."Wait for trigger" ("FF state") -> [w380]
    shift-right: [w372] -> _
    shift-left: TRUE ("decrement") -> [w373]
    stop <- _ stop-if-true
    n245 = feedback #27() -> (w377:bool)  [unwired: 1 in]
    n246 = call-poly <instrlib>:"Count Down.vi"("count in"=u8 2, "load"=w377, "decrement"=TRUE) -> ("terminal count"=w376:bool)  [unwired: 11 in, 1 out]
    n247 = feedback-in #27(w376) -> ()
    n248 = call "Adress counter.vi"("input valid"=w376, "Reset"=w373) -> ("output valid"=w375:bool, "Address"=w383:u32)  [unwired: 8 in]
    n249 = feedback #28() -> (w382:u32)  [unwired: 1 in]
    n250 = feedback-in #28(w383) -> ()
    n251 = case shown="\"Clear FF\"" w380 {
      selector: w380 -> [w390 w402 w421 w433]
      tunnel: w382 -> [_ _ w418 w430]
      tunnel: [w389 w407 w420 w432] -> w371
      tunnel: "Load FF" -> [w400 w406 _ _]
      tunnel: w375 -> [_ _ w411 _]
      tunnel: "Clear feedback buffers" -> [w396 w405 _ _]
      tunnel: [TRUE ("decrement") TRUE ("decrement") _ _] -> w372
      tunnel: "FF buffers manual" -> [w387 _ _ _]
      frame "Wait for trigger", Default {
        n252 = Select(t=FeedForwardState."Read FF" ("FF state"), s=w400, f=w390) -> (s? t:f=w397:T4)
        n253 = xnode ("Register Write")() -> ("Data"=w393:bool)  [unwired: 1 in, 1 out]
        n254 = xnode ("Register Write")() -> ("Data"=w394:bool)  [unwired: 1 in, 1 out]
        n255 = Select(t=FeedForwardState."Clear FF" ("FF state"), s=w396, f=w397) -> (s? t:f=w391:T4)
        n256 = Not(x=w394) -> (.not. x?=w392:bool)
        n257 = And(x=w393, y=w392) -> (x .and. y?=w388:bool)
        n258 = And(x=w387, y=w388) -> (x .and. y?=w386:bool)
        n259 = call <instrlib>:"Detect Rising Edge.vi"("signal"=w388) -> ("edge detected"=w385:bool)  [unwired: 14 in]
        n260 = Or(x=w386, y=w385) -> (x .or. y?=w384:bool)
        n261 = Select(t=w391, s=w384, f=w390) -> (s? t:f=w389:T4)
      }
      frame "Wait for reset" {
        n262 = Or(x=w405, y=w406) -> (x .or. y?=w404:bool)
        n263 = Select(t=w402, s=w404, f=FeedForwardState."Wait for trigger" ("FF state")) -> (s? t:f=w407:T4)
      }
      frame "Read FF" {
        w408 = fxp<+/-,32,14> 0.0 ("element")
        n264 = xnode ("Memory Method Node")("Address"=w418) -> ("Data"=w427:fxp<+/-,32,14>)  [unwired: 1 in, 1 out]
        n265 = xnode ("Memory Method Node")("Address"=w418) -> ("Data"=w419:fxp<+/-,32,14>)  [unwired: 1 in, 1 out]
        n266 = xnode ("Memory Method Node")("Address"=w418) -> ("Data"=w426:fxp<+/-,32,14>)  [unwired: 1 in, 1 out]
        n267 = xnode ("Memory Method Node")("Address"=w418) -> ("Data"=w417:fxp<+/-,32,14>)  [unwired: 1 in, 1 out]
        n268 = feedback #29() -> (w425:fxp<+/-,32,14>)  [unwired: 1 in]
        n269 = feedback-in #29(w427) -> ()
        n270 = feedback #30() -> (w416:fxp<+/-,32,14>)  [unwired: 1 in]
        n271 = feedback-in #30(w419) -> ()
        n272 = feedback #31() -> (w424:fxp<+/-,32,14>)  [unwired: 1 in]
        n273 = feedback-in #31(w426) -> ()
        n274 = feedback #32() -> (w415:fxp<+/-,32,14>)  [unwired: 1 in]
        n275 = feedback-in #32(w417) -> ()
        n276 = xnode ("Register Read")() -> ("Data"=w412:u16)  [unwired: 1 in, 1 out]
        n277 = Build Array(w408, w408, w425, w424, w416, w415) -> (w413:fxp<+/-,32,14>[])
        n278 = call "FormatDMAelement_6_elements.vi"("valid in"=w411, "factor"=w412, "Data in"=w413) -> ("valid out"=w409:bool, "Values"=w410:u64[])  [unwired: 7 in]
        n279 = case shown="True" w409 {
          tunnel: w410 -> [_ w428]
          frame False {
          }
          frame True {
            n280 = xnode ("FIFO Method Node")("Element"=w428, "Timeout"=0) -> ()  [unwired: 1 in, 2 out]
          }
        }
        n281 = Less?(x=w418, y=u32 40000) -> (x < y?=w422:bool)
        n282 = Select(t=w421, s=w422, f=FeedForwardState."Wait for reset" ("FF state")) -> (s? t:f=w420:T4)
        "Read FF address" <- w418
      }
      frame "Clear FF" {
        w431 = fxp<+/-,32,14> 0.0 ("Data")
        n283 = xnode ("Memory Method Node")("Address"=w430, "Data"=w431) -> ()  [unwired: 1 in, 1 out]
        n284 = xnode ("Memory Method Node")("Address"=w430, "Data"=w431) -> ()  [unwired: 1 in, 1 out]
        n285 = xnode ("Memory Method Node")("Address"=w430, "Data"=w431) -> ()  [unwired: 1 in, 1 out]
        n286 = xnode ("Memory Method Node")("Address"=w430, "Data"=w431) -> ()  [unwired: 1 in, 1 out]
        n287 = Less?(x=w430, y=u32 40000) -> (x < y?=w435:bool)
        n288 = Select(t=w433, s=w435, f=FeedForwardState."Wait for reset" ("FF state")) -> (s? t:f=w432:T4)
      }
    }
  }
  n289 = node-c288() -> (w18:T5)  [unwired: 1 in]
  n290 = timed-loop {
    timing: w18 -> [_]
    timing-out: [_] -> w17
    stop <- _ stop-if-true
    n291 = xnode "FPGA I/O Node"("IO Module\\AO Data Sync"="IO Module\\AO Data Sync") -> ()  [unwired: 1 in, 1 out]
  }
  n292 = node-c288() -> (w20:T5)  [unwired: 1 in]
  n293 = timed-loop {
    timing: w20 -> [_]
    timing-out: [_] -> w19
    stop <- _ stop-if-true
    n294 = xnode "FPGA I/O Node"("IO Module\\SPI Device"="IO Module\\SPI Device", "IO Module\\SPI Address"="IO Module\\SPI Address", "IO Module\\SPI Write Data"="IO Module\\SPI Write Data", "IO Module\\SPI Read"="IO Module\\SPI Read", "IO Module\\SPI Write"="IO Module\\SPI Write") -> ("IO Module\\SPI Idle"=→"IO Module\\SPI Idle":bool, "IO Module\\SPI Read Data"=→"IO Module\\SPI Read Data":u8)  [unwired: 7 in, 7 out]
  }
  n295 = node-c288(w28) -> ()
  n296 = node-c288(w21) -> ()
  n297 = node-c288(w23) -> ()
  n298 = node-c288(w10) -> ()
  n299 = node-c288(w8) -> ()
  n300 = node-c288(w26) -> ()
  n301 = node-c288(w2) -> ()
  n302 = node-c288(w6) -> ()
  n303 = node-c288(w17) -> ()
  n304 = node-c288(w13) -> ()
  n305 = node-c288(w19) -> ()
  n306 = node-c288(w15) -> ()
